vi "Start Sync.vi"(8 "error in (no error)":errorcluster, 11 "gRPC Server in":refnum<class "RouteGuide.lvclass">) -> (0 "error out":errorcluster, 3 "gRPC Server out":refnum<class "RouteGuide.lvclass">)   [LabVIEW 2019, in "Generated_server.lvlib" / "RouteGuide.lvclass"]
uses:
  RouteGuide.lvclass
  RouteGuide.lvclass/RouteGuide.ctl
  RPC Messages/routeguide_response.ctl
  RPC Messages/routeguide_Color.ctl
  Generated_server.lvlib
  <vilib>/gRPC/LabVIEW gRPC Library/grpc-lvsupport-release.lvlib
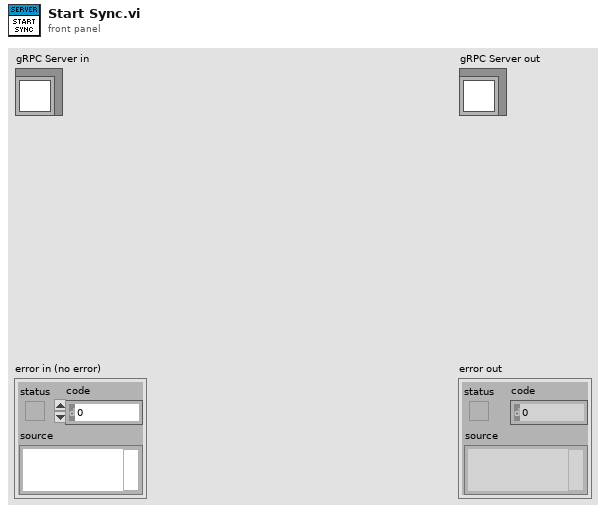
[diagram p1: front panel]
types:
  T1 = typedef "Generated_server.lvlib/routeguide_response.ctl" = cluster{"response_number":i32, "response_message":string, "response_color":T2}
  T2 = typedef "Generated_server.lvlib/routeguide_Color.ctl" = enum32{"RED", "GREEN", "BLUE"}
  T3 = typedef "Generated_server.lvlib/RouteGuide.lvclass/Server Internal UEs.ctl" = cluster{"RouteGuide UnaryMethod Internal UE":refnum<user-event>, "RouteGuide ServerStreamingMethod Internal UE":refnum<user-event>, "RouteGuide ClientStreamingMethod Internal UE":refnum<user-event>, "RouteGuide BidirectionalStreamingMethod Internal UE":refnum<user-event>}
  T4 = typedef "Generated_server.lvlib/RouteGuide.lvclass/Server gRPC UEs.ctl" = cluster{"RouteGuide UnaryMethod gRPC UE":refnum<user-event>, "RouteGuide ServerStreamingMethod gRPC UE":refnum<user-event>, "RouteGuide ClientStreamingMethod gRPC UE":refnum<user-event>, "RouteGuide BidirectionalStreamingMethod gRPC UE":refnum<user-event>}
  T5 = typedef "grpc-lvsupport-release.lvlib/grpcId.ctl" = u64
  T6 = typedef "Generated_server.lvlib/routeguide_request.ctl" = cluster{"request_number":i32, "request_message":string, "request_color":T2}
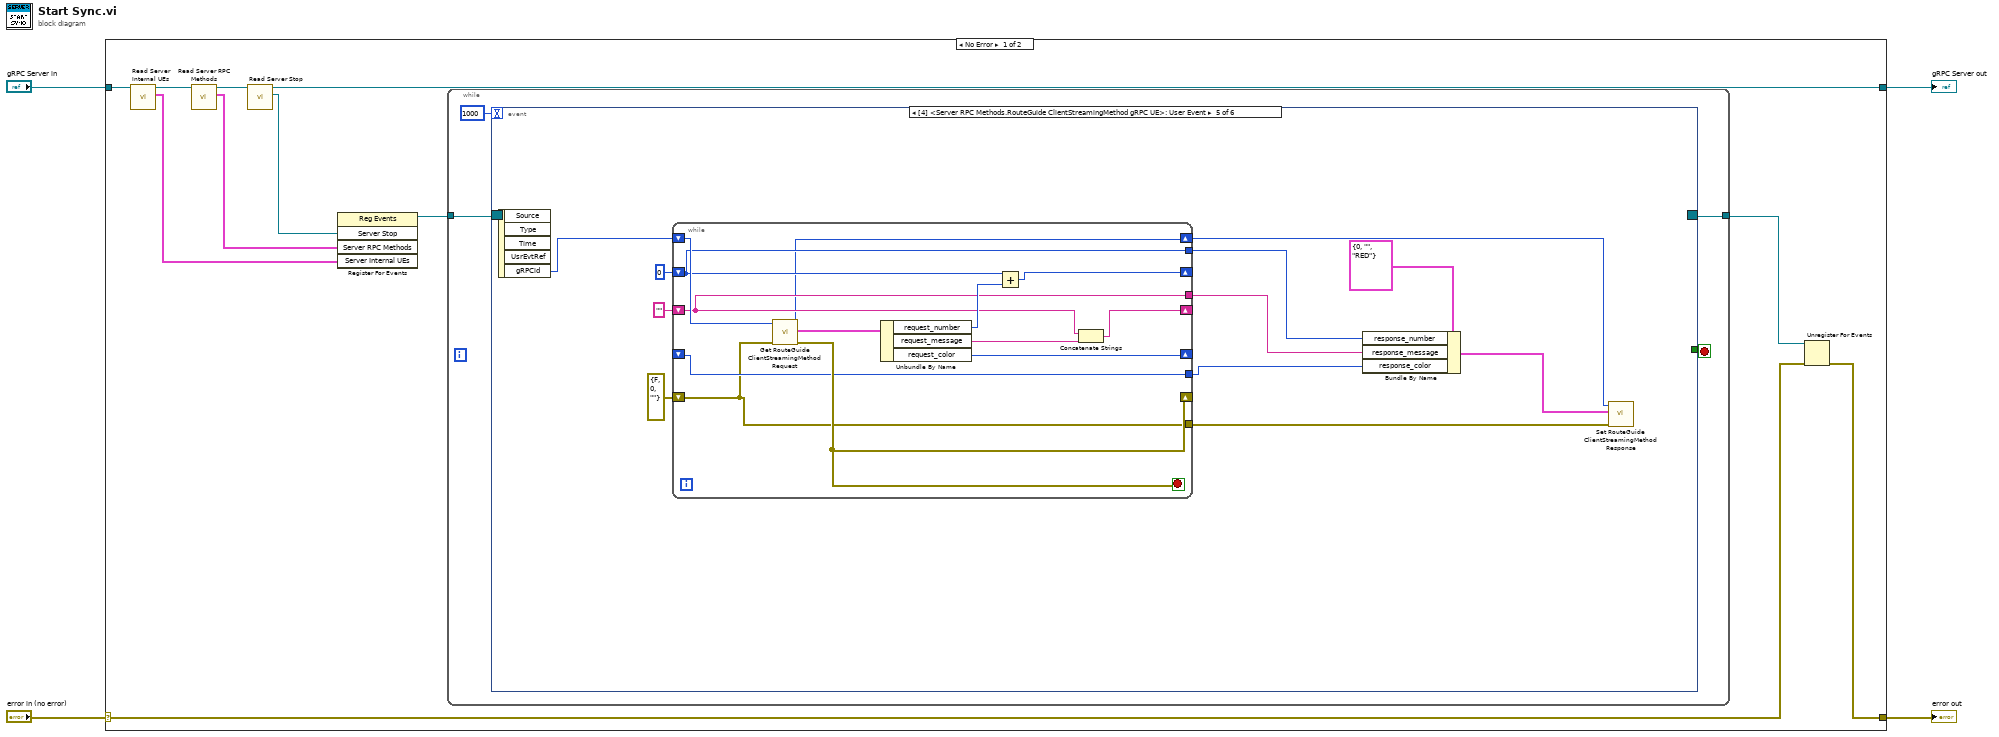
[diagram p0: block diagram]
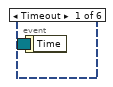
[diagram p2: hidden frame]
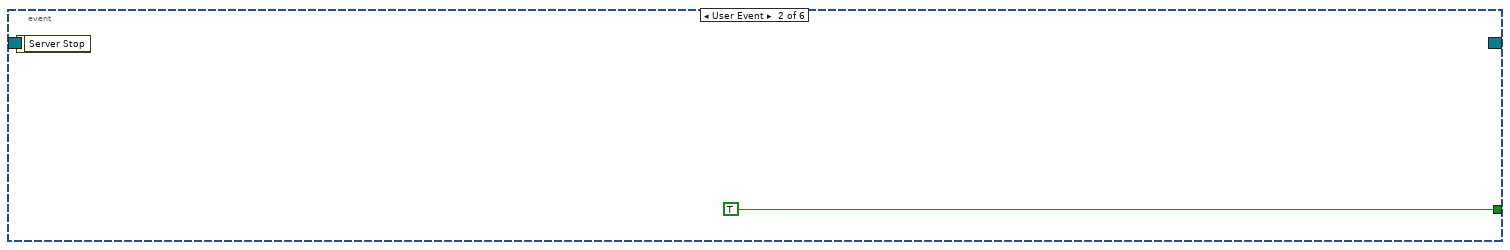
[diagram p3: hidden frame]
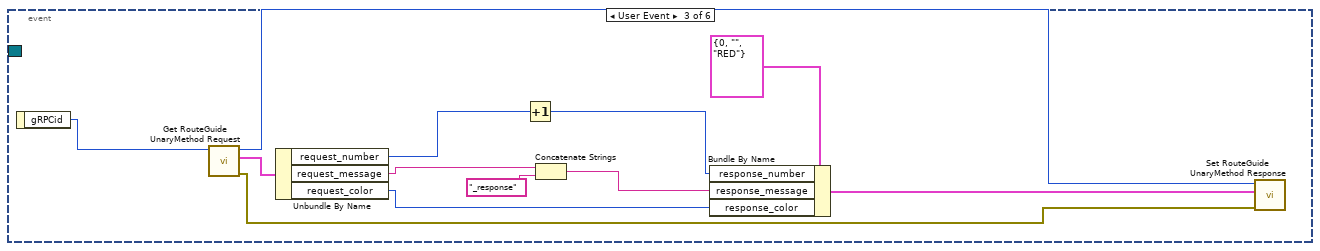
[diagram p4: hidden frame]
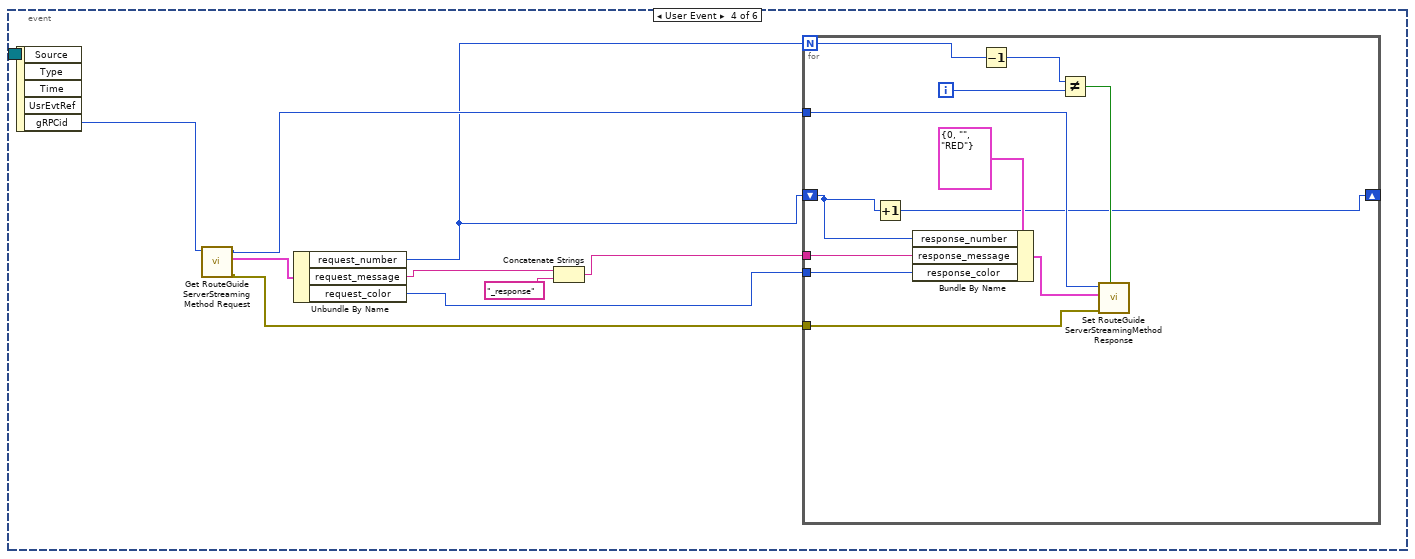
[diagram p5: hidden frame]
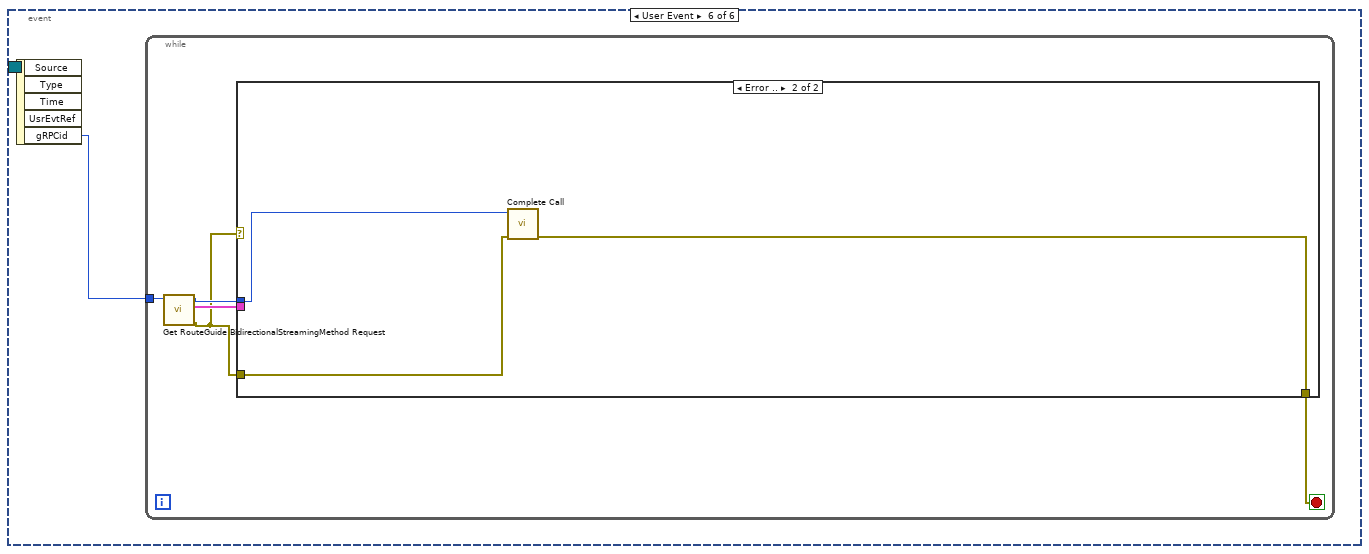
[diagram p6: hidden frame]
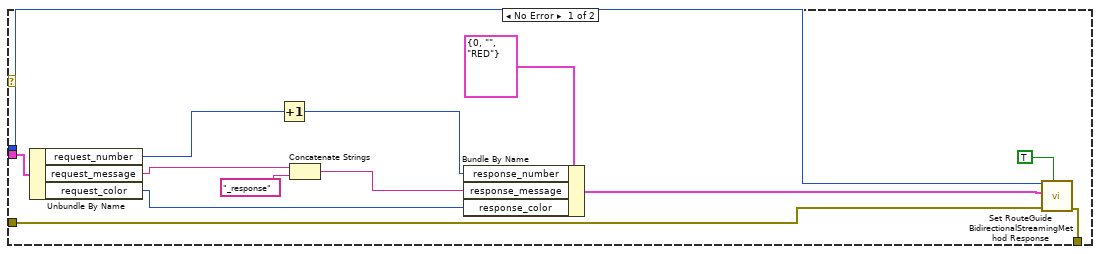
[diagram p7: hidden frame]
diagram:
  n1 = case shown="No Error" "error in (no error)" {
    selector: "error in (no error)" -> [w9 w101]
    tunnel: [w8 w101] -> w3
    tunnel: [w6 w100] -> w1
    tunnel: "gRPC Server in" -> [w15 w100]
    frame No Error {
      n2 = call "Read Server Internal UEs.vi"("SignalGeneratorService in"=w15) -> ("Server Internal UEs"=w13:T3, "SignalGeneratorService out"=w14:refnum<class "RouteGuide.lvclass">)  [unwired: 8 in, 1 out]
      n3 = call "Read Server RPC Methods.vi"("SignalGeneratorService in"=w14) -> ("Server RPC Methods"=w7:T4, "SignalGeneratorService out"=w12:refnum<class "RouteGuide.lvclass">)  [unwired: 8 in, 1 out]
      n4 = call-dynamic "Read Server Stop.vi"("iService in"=w12) -> ("Server Stop"=w5:refnum<user-event>, "iService out"=w6:refnum<class "RouteGuide.lvclass">)  [unwired: 8 in, 1 out]
      n5 = register-events(w5, w7, w13) -> (reference out=w11:refnum<event-registration>)  [unwired: 2 in, 1 out]
      n6 = while {
        tunnel: w11 -> [w19]
        tunnel: [w17] -> w10
        stop <- w18 stop-if-true
        n7 = event "RPC Methods Event Structure" shown="[4] <Server RPC Methods.RouteGuide ClientStreamingMethod gRPC UE>: User Event" {
          selector: w19 -> [_ _ _ _ _ _]
          dyn-events: [_ _ _ _ _ _] -> w17
          timeout: 1000 -> [_ _ _ _ _ _]
          tunnel: [_ TRUE _ _ _ _] -> w18
          event Timeout {
            n8 = event-data() -> ()  [unwired: 1 in, 1 out]
          }
          event User Event {
            n9 = event-data() -> ()  [unwired: 1 in, 1 out]
          }
          event User Event {
            n10 = event-data() -> ("gRPCid"=w32:T5)  [unwired: 1 in]
            n11 = call "Get RouteGuide UnaryMethod Request.vi"("gRPCid"=w32) -> ("error out"=w22:errorcluster, "Message Data"=w31:T6, "gRPCid out"=w21:T5)  [unwired: 8 in]
            n12 = Unbundle By Name(w31) -> ("request_number"=w30:i32, "request_message"=w29:string, "request_color"=w24:T2)
            n13 = Increment(x=w30) -> (x+1=w26:i32)
            n14 = Concatenate Strings(w29, "_response" ("string")) -> (w25:string)
            n15 = Bundle By Name(cluster=T1 {"response_number"=0, "response_message"="", "response_color"=enum."RED"} ("routeguide_response"), "response_number"=w26, "response_message"=w25, "response_color"=w24) -> (w23:T1)
            n16 = call "Set RouteGuide UnaryMethod Response.vi"("error in (no error)"=w22, "Message Data"=w23, "gRPCid in"=w21) -> ()  [unwired: 8 in, 1 out]
          }
          event User Event {
            n17 = event-data() -> ("gRPCid"=w38:T5)  [unwired: 1 in, 4 out]
            n18 = call "Get RouteGuide ServerStreamingMethod Request.vi"("gRPCid"=w38) -> ("error out"=w36:errorcluster, "Message Data"=w39:T6, "gRPCid out"=w37:T5)  [unwired: 8 in]
            n19 = Unbundle By Name(w39) -> ("request_number"=w33:i32, "request_message"=w41:string, "request_color"=w34:T2)
            n20 = Concatenate Strings(w41, "_response" ("string")) -> (w35:string)
            n21 = for {
              N: w33 -> [w51]
              tunnel: w37 -> [w53]
              tunnel: w36 -> [w52]
              tunnel: w35 -> [w47]
              tunnel: w34 -> [w46]
              shift-right: [w42] -> _
              shift-left: w33 -> [w43]
              i -> [w49]
              n22 = Increment(x=w43) -> (x+1=w42:i32)
              n23 = Bundle By Name(cluster=T1 {"response_number"=0, "response_message"="", "response_color"=enum."RED"} ("routeguide_response"), "response_number"=w43, "response_message"=w47, "response_color"=w46) -> (w45:T1)
              n24 = Decrement(x=w51) -> (x-1=w50:i32)
              n25 = Not Equal?(x=w50, y=w49) -> (x != y?=w48:bool)
              n26 = call "Set RouteGuide ServerStreamingMethod Response.vi"("Streaming? (F)"=w48, "error in (no error)"=w52, "Message Data"=w45, "gRPCid in"=w53) -> ()  [unwired: 7 in, 1 out]
            }
          }
          event User Event {
            n27 = event-data() -> ("gRPCid"=w64:T5)  [unwired: 1 in, 4 out]
            n28 = while {
              shift-right: [w76] -> _
              shift-left: errorcluster {"status"=FALSE, "code"=0, "source"=""} ("error out") -> [w65]
              shift-right: [w73] -> _
              shift-left: 0 -> [w72]
              tunnel: [w72] -> w59
              shift-right: [w70] -> _
              shift-left: "" -> [w69]
              tunnel: [w69] -> w58
              shift-right: [w68] -> _
              shift-left: _ -> [w67]
              tunnel: [w67] -> w54
              shift-right: [w66] -> w56
              shift-left: w64 -> [w77]
              tunnel: [w65] -> w55
              stop <- w76 stop-if-true
              n29 = call "Get RouteGuide ClientStreamingMethod Request.vi"("error in (no error)"=w65, "gRPCid"=w77) -> ("error out"=w76:errorcluster, "Message Data"=w75:T6, "gRPCid out"=w66:T5)  [unwired: 7 in]
              n30 = Unbundle By Name(w75) -> ("request_number"=w74:i32, "request_message"=w71:string, "request_color"=w68:T2)
              n31 = Add(x=w72, y=w74) -> (x+y=w73:i32)
              n32 = Concatenate Strings(w69, w71) -> (w70:string)
            }
            n33 = Bundle By Name(cluster=T1 {"response_number"=0, "response_message"="", "response_color"=enum."RED"} ("routeguide_response"), "response_number"=w59, "response_message"=w58, "response_color"=w54) -> (w57:T1)
            n34 = call "Set RouteGuide ClientStreamingMethod Response.vi"("error in (no error)"=w55, "Message Data"=w57, "gRPCid in"=w56) -> ()  [unwired: 8 in, 1 out]
          }
          event User Event {
            n35 = event-data() -> ("gRPCid"=w78:T5)  [unwired: 1 in, 4 out]
            n36 = while {
              tunnel: w78 -> [w83]
              stop <- w81 stop-if-true
              n37 = call "Get RouteGuide BidirectionalStreamingMethod Request.vi"("gRPCid"=w83) -> ("error out"=w79:errorcluster, "Message Data"=w80:T6, "gRPCid out"=w82:T5)  [unwired: 8 in]
              n38 = case shown="Error .." w79 {
                tunnel: w82 -> [w89 w99]
                tunnel: w79 -> [w87 w98]
                tunnel: [w86 w97] -> w81
                tunnel: w80 -> [w84 _]
                frame No Error {
                  n39 = Unbundle By Name(w84) -> ("request_number"=w96:i32, "request_message"=w95:string, "request_color"=w90:T2)
                  n40 = Increment(x=w96) -> (x+1=w92:i32)
                  n41 = Concatenate Strings(w95, "_response" ("string")) -> (w91:string)
                  n42 = Bundle By Name(cluster=T1 {"response_number"=0, "response_message"="", "response_color"=enum."RED"} ("routeguide_response"), "response_number"=w92, "response_message"=w91, "response_color"=w90) -> (w88:T1)
                  n43 = call "Set RouteGuide BidirectionalStreamingMethod Response.vi"("Streaming? (F)"=TRUE, "error in (no error)"=w87, "Message Data"=w88, "gRPCid in"=w89) -> ("error out"=w86:errorcluster)  [unwired: 7 in]
                }
                frame Error {
                  n44 = call <vilib>:"Complete Call.vi"("gRPCid"=w99, "error in"=w98) -> ("error out"=w97:errorcluster)  [unwired: 8 in]
                }
              }
            }
          }
        }
      }
      n45 = Unregister For Events(event registration refnum=w10, error in=w9) -> (error out=w8:errorcluster)
    }
    frame Error {
    }
  }
  "error out" <- w3
  "gRPC Server out" <- w1
